vi "Thumbstick Read.vi"(0 "Arduino Resource":T1={"VISA resource"="", "Board Type"=enum."Arduino Uno", "Connection Type"=enum."USB / Serial", "Bytes Per Packet (15)"=15}, 7 "Thumbstick Data":T5, 11 "error in":errorcluster) -> (4 "Arduino Resource":T1={"VISA resource"="", "Board Type"=enum."Arduino Uno", "Connection Type"=enum."USB / Serial", "Bytes Per Packet (15)"=15}, 6 "Horizontal Axis":dbl, 8 "Vertical Axis":dbl, 10 "Select (Active Low)":dbl, 15 "error out":errorcluster)   [LabVIEW 2011, in "LabVIEW Interface for Arduino.lvlib"]
doc: "Read thumbstick values from the Arduino."
uses:
  LabVIEW Interface for Arduino.lvlib
  Private/Type Defs/Analog Pin.ctl
  Private/Type Defs/Digital Pin.ctl
  Private/Type Defs/Arduino Resource.ctl
  Private/Type Defs/Board Type.ctl
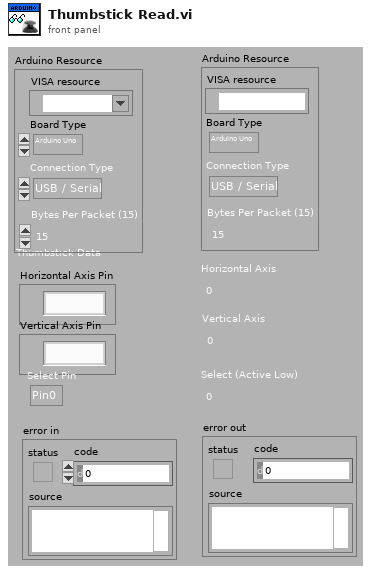
[diagram p1: front panel]
types:
  T1 = typedef "LabVIEW Interface for Arduino.lvlib/Arduino Resource.ctl" = cluster{"VISA resource":refnum<visa-resource-name>, "Board Type":T2, "Connection Type":enum8{"USB / Serial"}, "Bytes Per Packet (15)":u8}
  T2 = typedef "LabVIEW Interface for Arduino.lvlib/Board Type.ctl" = enum16{"Arduino Uno", "Dimuelanove w/Atmega 328", "Mega 2560", "Chipkit Uno32", "Chipkit Max32"}
  T3 = typedef "LabVIEW Interface for Arduino.lvlib/Analog Pin.ctl" = enum8{"AI_0", "AI_1", "AI_2", "AI_3", "AI_4", "AI_5", "AI_6", "AI_7", "AI_8", "AI_9", "AI_10", "AI_11", "AI_12", "AI_13", "AI_14", "AI_15"}
  T4 = typedef "LabVIEW Interface for Arduino.lvlib/Digital Pin.ctl" = enum8{"Pin0", "Pin1", "Pin2", "Pin3", "Pin4", "Pin5", "Pin6", "Pin7", "Pin8", "Pin9", "Pin10", "Pin11", "Pin12", "Pin13"}
  T5 = cluster{"Horizontal Axis Pin":T3, "Vertical Axis Pin":T3, "Select Pin":T4}
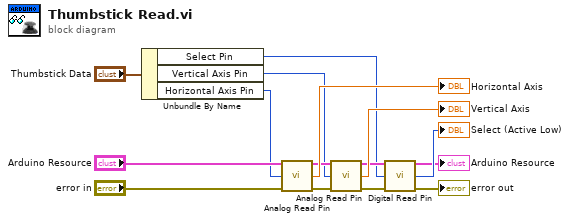
[diagram p0: block diagram]
diagram:
  n1 = Unbundle By Name("Thumbstick Data") -> ("Select Pin"=w3:T4, "Vertical Axis Pin"=w2:T3, "Horizontal Axis Pin"=w1:T3)
  n2 = call "Analog Read Pin.vi"("Arduino Resource"="Arduino Resource", "Analog Pin"=w1, "error in"="error in") -> ("Arduino Resource"=w7:T1, "Voltage"=→"Horizontal Axis":dbl, "error out"=w14:errorcluster)  [unwired: 10 in]
  n3 = call "Analog Read Pin.vi"("Arduino Resource"=w7, "Analog Pin"=w2, "error in"=w14) -> ("Arduino Resource"=w6:T1, "Voltage"=→"Vertical Axis":dbl, "error out"=w13:errorcluster)  [unwired: 10 in]
  n4 = call "Digital Read Pin.vi"("Arduino Resource"=w6, "Digital I/O Pin (0)"=w3, "error in"=w13) -> ("Arduino Resource"=→"Arduino Resource":T1, "Value"=→"Select (Active Low)":u8, "error out"=→"error out":errorcluster)  [unwired: 10 in]
